vi "SV TDMS Write Order Level Components (1xM).vi"(0 "tdms file":refnum<k34>, 2 "write mode":u16(ring) items=["Append", "New group", "Overwrite"], 5 "group name in":string, 7 "channel name in":string="Channel0", 9 "order component":cluster{"X":dbl[], "Y":dbl[]}[](array[cluster]), 11 "error in":errorcluster, 12 "component":T1=32 items=["Magnitude"=32, "Phase"=33, "Real"=34, "Imaginary"=35, "Coherence"=36, "Unknown"=99], 13 "spectrum info":T2 {"x-axis units" items=["Time (s)"=0, "Frequency-CB (Hz)"=1, "Frequency-CPB (Hz)"=1248, "Frequency-Arbitrary (Hz)"=2357, "Quefrency (s)"=2, "Revolutions (rev)"=3, "Order"=4, "Speed (RPM)"=11, "Speed (rad/s)"=21, "Index"=65535]; "weighting filter" items=["Linear", "A-weighting", "B-weighting", "C-weighting", "ITU-R 468-4", "Dolby", "CCITT", "C-message", "Wb", "Wc", "Wd", "We", "Wf", "Wh", "Wj", "Wk", "Wm", "AES17 20 kHz lowpass", "AES17 40 kHz lowpass", "AES17 20 kHz highpass", "AES17 40 kHz highpass"]; "dB reference [EU]" format="%.2f"; "engineering units" items=["custom..."=0, "V"=1, "A"=21, "C"=30, "pC"=31, "s"=32, "-"=29, "Pa"=2, "N"=20, "g"=3, "m/s^2"=4, "m/s"=5, "m"=6, "mm/s"=12, "mm"=13, "micron/s"=14, "micron"=15, "in/s^2"=7, "in/s"=8, "in"=9, "mil/s"=10, "mil"=11, "rad/s^2"=16, "rad/s"=17, "rad"=18, "deg/s^2"=26, "deg/s"=27, "deg"=28, "RPM"=22, "cycle/s^2"=23, "Hz"=24, "cycle"=25, "strain"=19]; "spectral info"."window" items=["None "=0, "Hanning"=1, "Hamming"=2, "Blackman-Harris"=3, "Exact Blackman"=4, "Blackman"=5, "Flat Top"=6, "4 Term B-Harris "=7, "7 Term B-Harris"=8, "Low Sidelobe"=9, "Force - Exponential"=10, "Gaussian"=62]}) -> (4 "tdms file out":refnum<k34>, 6 "group name out":string, 8 "channel names out":string[](array[string]), 15 "error out":errorcluster)   [LabVIEW 2017]
doc: "Writes data to the specified .tdms file in a format specific to the polymorphic instance. Wire data to the <B>scaled signal [EU]</B> input to determine the polymorphic instance to use or manually select the instance."
uses:
  <vilib>/addons/_NISVFA/_Shared subVIs/Controls/svc_Spectrum Info.ctl
  <vilib>/addons/_NISVFA/_Shared subVIs/Controls/svc_X-Axis Units.ctl
  <vilib>/addons/_NISVFA/_Shared subVIs/Controls/svc_Spectrum Type.ctl
  <vilib>/addons/_NISVFA/_Shared subVIs/Controls/svc_Engineering Units Text Ring.ctl
  <vilib>/addons/_NISVFA/_Shared subVIs/Controls/svc_Weighting Filter Text Ring.ctl
  <vilib>/addons/_NISVFA/_Shared subVIs/Controls/svc_Complimentary Spectrum Units.ctl
  <vilib>/addons/_NISVFA/_Shared subVIs/Controls/NI Spectrum Component.ctl
  <vilib>/addons/_NISVFA/_Shared subVIs/Controls/LV Datatypes.ctl
  <vilib>/addons/_NISVFA/_Shared subVIs/Controls/NI Function Type.ctl
  <vilib>/addons/_NISVFA/_Shared subVIs/Controls/NI Channel Properties.ctl
  <vilib>/addons/_NISVFA/_Shared subVIs/Controls/SV Channel Properties.ctl
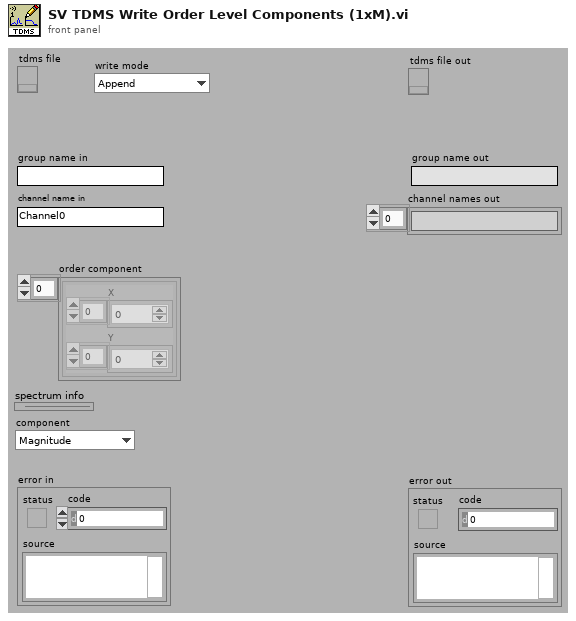
[diagram p1: front panel]
types:
  T1 = typedef "NI Spectrum Component.ctl" = u16
  T2 = typedef "svc_Spectrum Info.ctl" = cluster{"channel name":string, "description":string, "x-axis units":T3, "spectral info":cluster{"spectrum type":T4, "linear/dB":enum16{"linear", "dB"}, "window":u16, "window size":i32, "FFT size":i32}, "engineering units":T5, "custom label":string, "dB reference [EU]":dbl, "peak units":enum16{"rms", "peak", "peak-peak"}, "weighting filter":T6, "spectral density?":bool, "unit label":string, "spectrum skewed?":bool, "complimentary spectrum units":T7}
  T3 = typedef "svc_X-Axis Units.ctl" = u16
  T4 = typedef "svc_Spectrum Type.ctl" = enum16{"FFT Spectrum [complex]", "Amplitude [Magnitude]", "Power [Magnitude^2]", "Cross Spectrum [complex]", "Frequency Response [Complex]"}
  T5 = typedef "svc_Engineering Units Text Ring.ctl" = u16
  T6 = typedef "svc_Weighting Filter Text Ring.ctl" = u16
  T7 = typedef "svc_Complimentary Spectrum Units.ctl" = enum16{"none", "radians", "degrees", "cycles", "imaginary"}
  T8 = typedef "SV Channel Properties.ctl" = u16
  T9 = typedef "NI Channel Properties.ctl" = u16
  T10 = typedef "NI Function Type.ctl" = u16
  T11 = typedef "LV Datatypes.ctl" = i32
  T12 = typedef "NI Function SubType.ctl" = u16
  T13 = cluster{"function type":T10, "function subtype":T12, "X-domain":T3}
  T14 = cluster{"X-axis label":string, "X-unit string":string, "Y-axis label":string, "Y-unit string":string}
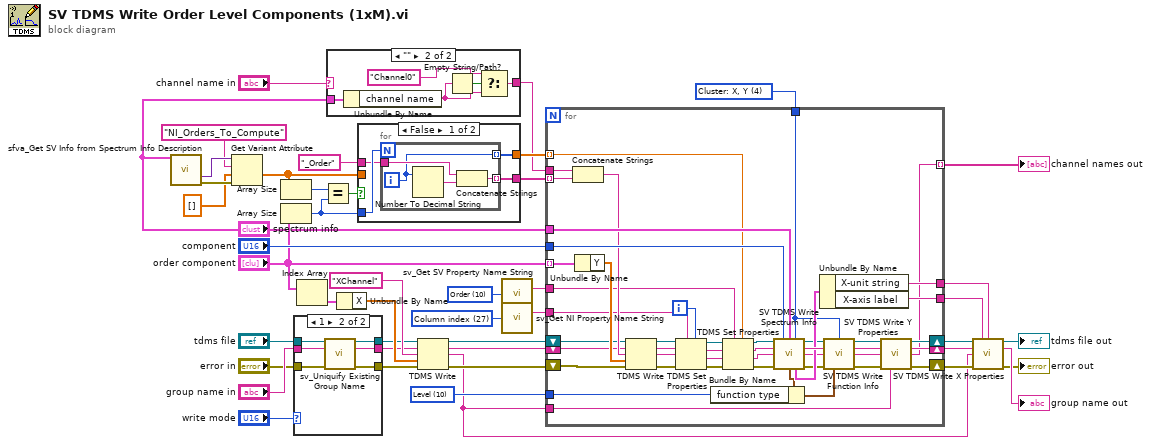
[diagram p0: block diagram]
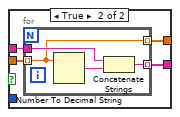
[diagram p4: hidden frame]
diagram:
  w18 = T8 10 items=["Engineering units", "Custom unit label", "Weighting filter", "Pregain", "Octave standard", "Octave bandwidth", "Octave low band", "Octave high band", "Spectrum skewed", "Samples / revolution", "Order"] ("property")
  w37 = T9 27 items=["Channel name", "Channel description", "Axis label", "Unit string", "Waveform X-axis label", "Waveform X-axis unit string", "x0", "dx", "Number of samples", "X channel", "Filter settled", "dB reference", "Window", "Window parameter", "Window size", "FFT size", "Peak units", "Spectrum type", "Magnitude scale", "Spectral density", "Sensor sensitivity (mV/EU)", "X-axis dimension", "LabVIEW datatype", "Function type", "Function subtype", "X values", "Independent channel", "Column index"] ("property")
  w43 = T10 10 items=["Signal"=0, "Speed"=3, "Level"=10, "Octave Spectrum"=20, "FFT Spectrum"=30, "Cross Spectrum"=40, "Frequency Response"=50, "Ratio"=6, "Count"=7] ("function type")
  w44 = T11 4 items=["String: abc"=-2, "Boolean: True or False"=-1, "Scalar: y"=0, "Array: Y"=1, "Waveform: t0, dt, Y, variant"=2, "Cluster: x0, dx, Y"=3, "Cluster: X, Y"=4, "Waterfall"=5, "Colormap"=6] ("LabVIEW datatype")
  n1 = call <vilib>:"sfva_Get SV Info from Spectrum Info Description.vi"("spectrum info"="spectrum info") -> ("SV Info"=w12:variant, "error out"=w13:errorcluster)  [unwired: 10 in, 3 out]
  n2 = Get Variant Attribute(Variant=w12, name="NI_Orders_To_Compute", default value (empty Variant)=dbl[] [] ("orders to compute"), error in=w13) -> (value=w10:dbl[])  [unwired: 3 out]
  n3 = Array Size(array=w10) -> (size(s)=w39:i32)
  n4 = Array Size(array="order component") -> (size(s)=w40:i32)
  n5 = case shown="1" "write mode" {
    tunnel: [w48 w53] -> w2
    tunnel: [w46 w49] -> w5
    tunnel: "group name in" -> [w46 w50]
    tunnel: [w47 w51] -> w1
    tunnel: "error in" -> [w47 w52]
    tunnel: "tdms file" -> [w48 w54]
    frame 0, Default {
    }
    frame 1 {
      n6 = call <vilib>:"sv_Uniquify Existing Group Name.vi"("tdms file ref"=w54, "group name"=w50, "error in"=w52) -> ("tdms file out"=w53:refnum<k34>, "unique group"=w49:string, "error out"=w51:errorcluster)  [unwired: 10 in]
    }
  }
  n7 = Index Array(array="order component") -> (element=w35:cluster{"X":dbl[], "Y":dbl[]})  [unwired: 1 in]
  n8 = Equal?(x=w39, y=w40) -> (x = y?=w41:bool)
  n9 = case shown="\"\"" "channel name in" {
    selector: "channel name in" -> [w55 _]
    tunnel: "spectrum info" -> [_ w59]
    tunnel: [w55 w57] -> w15
    frame Default {
    }
    frame "" {
      n10 = Unbundle By Name(w59) -> ("channel name"=w58:string)
      n11 = Empty String/Path?(string/path=w58) -> (empty?=w60:bool)
      n12 = Select(t="Channel0", s=w60, f=w58) -> (s? t:f=w57:string)
    }
  }
  n13 = Unbundle By Name(w35) -> ("X"=w31:dbl[])
  n14 = case shown="False" w41 {
    tunnel: [w63 w71] -> w38
    tunnel: w40 -> [w64 _]
    tunnel: w10 -> [_ w72]
    tunnel: [w62 w70] -> w19
    tunnel: "_Order" ("string") -> [w61 w69]
    frame False {
      n15 = for {
        N: w64 -> [_]
        tunnel: w61 -> [w67]
        tunnel: [w66] -> w63 mode=indexing
        tunnel: [w65] -> w62 mode=indexing
        i -> [w65]
        n16 = Number To Decimal String(number=w65) -> (decimal integer string=w68:string)  [unwired: 1 in]
        n17 = Concatenate Strings(w67, w68) -> (w66:string)
      }
    }
    frame True {
      n18 = for {
        tunnel: w72 -> [w73] mode=indexing
        tunnel: [w75] -> w71 mode=indexing
        tunnel: w69 -> [w74]
        tunnel: [w73] -> w70 mode=indexing
        n19 = Number To Decimal String(number=w73) -> (decimal integer string=w76:string)  [unwired: 1 in]
        n20 = Concatenate Strings(w74, w76) -> (w75:string)
      }
    }
  }
  n21 = TDMS Write(0:w2, 5:w5, 7:"XChannel", 9:w31, 11:w1) -> (4:w34:refnum<k34>, 6:w33:string, 8:w20:string, 15:w32:errorcluster)  [unwired: 1 in]
  n22 = call <vilib>:"sv_Get SV Property Name String.vi"("property"=w18) -> ("TDMS property name"=w17:string)  [unwired: 13 in, 1 out]
  n23 = call <vilib>:"sv_Get NI Property Name String.vi"("property"=w37) -> ("TDMS property name"=w29:string)  [unwired: 13 in, 1 out]
  n24 = for {
    shift-right: [w92] -> w22
    shift-left: w32 -> [w102]
    shift-right: [w91] -> w25
    shift-left: w33 -> [w103]
    shift-right: [w90] -> w26
    shift-left: w34 -> [w104]
    tunnel: "order component" -> [w122] mode=indexing
    tunnel: "spectrum info" -> [w121]
    tunnel: "component" -> [w120]
    tunnel: w44 -> [w77]
    tunnel: w43 -> [w114]
    tunnel: w38 -> [w105] mode=indexing
    tunnel: w29 -> [w99]
    tunnel: [w94] -> w28
    tunnel: [w93] -> w27
    tunnel: w20 -> [w101]
    tunnel: w19 -> [w80] mode=indexing
    tunnel: w17 -> [w81]
    tunnel: w15 -> [w79]
    tunnel: [w78] -> w42 mode=indexing
    i -> [w98]
    n25 = Concatenate Strings(w79, w105) -> (w113:string)
    n26 = Unbundle By Name(w122) -> ("Y"=w119:dbl[])
    n27 = TDMS Write(0:w104, 5:w103, 7:w113, 9:w119, 11:w102) -> (4:w97:refnum<k34>, 6:w96:string, 8:w95:string, 15:w100:errorcluster)  [unwired: 1 in]
    n28 = TDMS Set Properties(5:w98, 7:w99, 8:w100, 9:w95, 10:w96, 11:w97) -> (0:w89:errorcluster, 1:w88:string, 2:w87:string, 3:w86:refnum<k34>)
    n29 = TDMS Set Properties(5:w80, 7:w81, 8:w89, 9:w88, 10:w87, 11:w86) -> (0:w82:errorcluster, 1:w83:string, 2:w84:string, 3:w85:refnum<k34>)
    n30 = call <vilib>:"SV TDMS Write Spectrum Info.vi"("tdms file"=w85, "spectrum component"=w120, "spectrum info"=w121, "LabVIEW datatype"=w77, "group name in"=w84, "channel name in"=w83, "error in"=w82) -> ("tdms file out"=w112:refnum<k34>, "group name out"=w118:string, "channel name out"=w111:string, "function info"=w116:T13, "unit info"=w117:T14, "error out"=w110:errorcluster)  [unwired: 3 in]
    n31 = Bundle By Name(cluster=w116, "function type"=w114) -> (w115:T13)
    n32 = Unbundle By Name(w117) -> ("X-unit string"=w94:string, "X-axis label"=w93:string)
    n33 = call <vilib>:"SV TDMS Write Function Info.vi"("tdms file in"=w112, "function info"=w115, "LabVIEW datatype"=w77, "group name"=w118, "channel name"=w111, "error in (no error)"=w110) -> ("tdms file out"=w106:refnum<k34>, "group name out"=w107:string, "channel name out"=w108:string, "error out"=w109:errorcluster)  [unwired: 6 in]
    n34 = call <vilib>:"SV TDMS Write Y Properties.vi"("tdms file"=w106, "group name"=w107, "channel name"=w108, "error in (no error)"=w109, "xchannel name"=w101) -> ("tdms file out"=w90:refnum<k34>, "group name"=w91:string, "channel name"=w78:string, "error out"=w92:errorcluster)  [unwired: 7 in]
  }
  "channel names out" <- w42
  n35 = call <vilib>:"SV TDMS Write X Properties.vi"("tdms file in"=w26, "X-axis label"=w27, "X-unit string"=w28, "group name"=w25, "channel name"=w20, "error in"=w22) -> ("tdms file out"=→"tdms file out":refnum<k34>, "group name"=→"group name out":string, "error out"=→"error out":errorcluster)  [unwired: 6 in, 1 out]
